vi "MCSPhotonCountingWriter.vi"(4 "ErrorIn":errorcluster, 5 "UDPResponse":string, 6 "MPDUnitID":T1=enum."MPD#04", 7 "PhotonCountingChannelMap":T2[](array[typedef])=[enum."WVOnline", enum."Unassigned", enum."Unassigned", enum."Unassigned", enum."Unassigned", enum."Unassigned", enum."Unassigned", enum."Unassigned", enum."WVOffline", enum."Unassigned", enum."Unassigned", enum."Unassigned"]) -> (0 "ErrorOut":errorcluster, 3 "ByteArray":u8[](array[numeric])=[64, 55, 34, 184, 91, 157, 14, 129, 0, 12, 0, 0, 0, 0, 0, 0, 1, 2, 3, 4, 5, 6, 0, 0, 80, 77, 30, 154, 10, 0, 46, 190, 4, 8, 0, 0, 0, 48, 0, 0, 0, 48, 0, 0, 0, 48, 0, 0, 0, 48, 0, 0, 0, 48, 171, 206, 4, 8, 0, 0, 0, 48, 0, 0, 0, 48, 0, 0, 0, 48, 0, 0, 0, 48, 0, 0, 0, 48, 255, 255, 255, 255, 13, 10])   [LabVIEW 2012]
uses:
  MCSPhotonCountingMap.ctl
  MPDUnitID.ctl
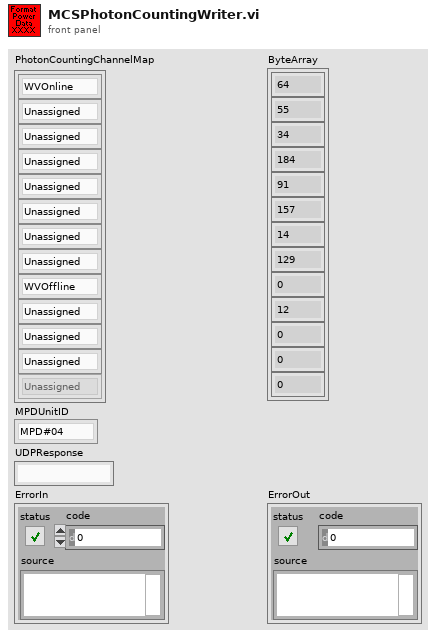
[diagram p1: front panel]
types:
  T1 = typedef "MPDUnitID.ctl" = enum8{"Unknown", "MPD#01", "MPD#02", "MPD#03", "MPD#04", "MPD#05"}
  T2 = typedef "MCSPhotonCountingMap.ctl" = enum8{"Unassigned", "Unknown", "WVOnline", "WVOnlineLow", "WVOffline", "WVOfflineLow", "O2Online", "O2OnlineLow", "O2Offline", "O2OfflineLow", "O2OnlineMol", "O2OnlineMolLow", "O2OnlineComb", "O2OnlineCombLow", "O2OfflineMol", "O2OfflineMolLow", "O2OfflineComb", "O2OfflineCombLow", "HSRLMol", "HSRLMolLow", "HSRLComb", "HSRLCombLow"}
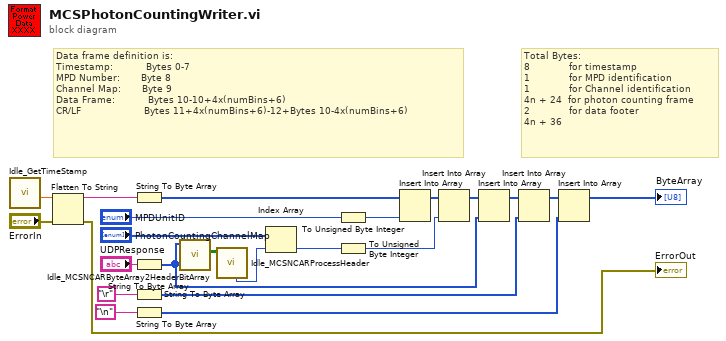
[diagram p0: block diagram]
diagram:
  # "Total Bytes:\n8             for timestamp\n1             for MPD identification\n1             for Channel identification\n4n + 24  for photon counting frame\n2             for data footer\n4n + 36"
  # "Data frame definition is:\nTimestamp:           Bytes 0-7\nMPD Number:       Byte 8\nChannel Map:       Byte 9\nData Frame:           Bytes 10-10+4x(numBins+6)\nCR/LF                     Bytes 11+4x(numBins+6)-12+Bytes 10-4x(numBins+6)"
  n1 = call "Idle_GetTimeStamp.vi"() -> ("Fractional Hours"=w18:dbl)  [unwired: 11 in]
  n2 = Flatten To String(anything=w18, error in (no error)="ErrorIn") -> (data string=w19:string, error out=→"ErrorOut":errorcluster)  [unwired: 2 in, 1 out]
  n3 = String To Byte Array(string=w19) -> (unsigned byte array=w6:u8[])
  n4 = String To Byte Array(string="UDPResponse") -> (unsigned byte array=w1:u8[])
  n5 = String To Byte Array(string="\r") -> (unsigned byte array=w13:u8[])
  n6 = String To Byte Array(string="\n") -> (unsigned byte array=w20:u8[])
  n7 = call "Idle_MCSNCARByteArray2HeaderBitArray.vi"("Input Byte Array"=w1) -> ("Header Array"=w5:bool[][])  [unwired: 9 in, 1 out]
  n8 = call "Idle_MCSNCARProcessHeader.vi"("Array"=w5) -> ("Channel"=w3:u32)  [unwired: 4 in, 6 out]
  n9 = Index Array(array="PhotonCountingChannelMap", index=w3) -> (element=w2:T2)
  n10 = To Unsigned Byte Integer(number="MPDUnitID") -> (unsigned 8bit integer=w10:u8)
  n11 = To Unsigned Byte Integer(number=w2) -> (unsigned 8bit integer=w17:u8)
  n12 = Insert Into Array(array=w6, new element=w10) -> (w7:u8[])  [unwired: 1 in]
  n13 = Insert Into Array(array=w7, new element=w17) -> (w16:u8[])  [unwired: 1 in]
  n14 = Insert Into Array(array=w16, new element=w1) -> (w15:u8[])  [unwired: 1 in]
  n15 = Insert Into Array(array=w15, new element=w13) -> (w14:u8[])  [unwired: 1 in]
  n16 = Insert Into Array(array=w14, new element=w20) -> (→"ByteArray":u8[])  [unwired: 1 in]
